vi "关闭文件.vi"(8 "error in (no error)":errorcluster caption="错误输入（无错误）", 11 "配置文件- 输入":refnum<class "配置文件-.lvclass">) -> (0 "error out":errorcluster caption="错误输出", 3 "配置文件- 输出":refnum<class "配置文件-.lvclass">)   [LabVIEW 2017, in "项目开发助手.lvlib" / "模板-配置文件相关.lvlib" / "配置文件-.lvclass"]
uses:
  <vilib>/Utility/config.llb/NI_LVConfig.lvlib
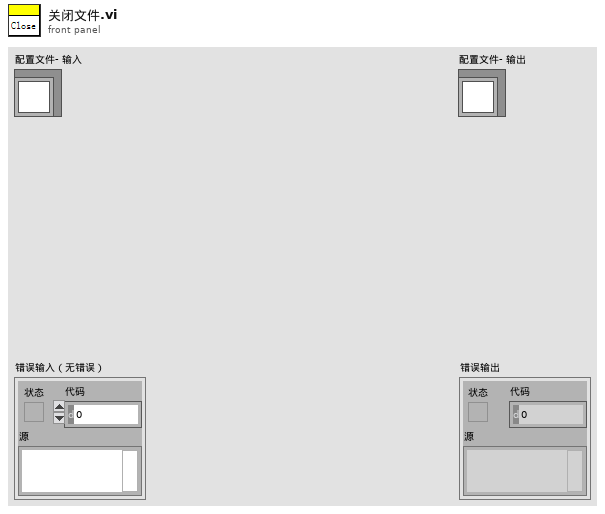
[diagram p1: front panel]
types:
  T1 = typedef "NI_LVConfig.lvlib/Config Data RefNum.ctl" = refnum<k1>
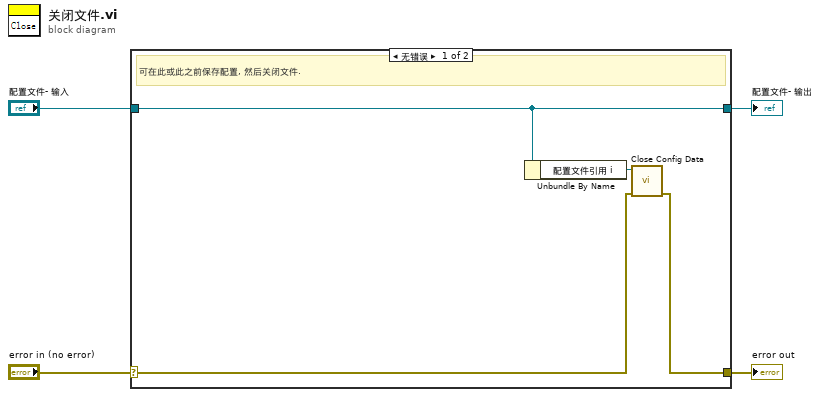
[diagram p0: block diagram]
diagram:
  n1 = case shown="无错误" "error in (no error)" {
    selector: "error in (no error)" -> [w6 w10]
    tunnel: [w5 w10] -> w3
    tunnel: [w8 w9] -> w1
    tunnel: "配置文件- 输入" -> [w8 w9]
    frame No Error {
      # "可在此或此之前保存配置, 然后关闭文件."
      n2 = Unbundle By Name(w8) -> ("配置文件引用 i"=w7:T1)
      n3 = call <vilib>:"Close Config Data.vi"("error in (no error)"=w6, "refnum"=w7) -> ("error out"=w5:errorcluster)  [unwired: 8 in, 1 out]
    }
    frame Error {
    }
  }
  "error out" <- w3
  "配置文件- 输出" <- w1
